vi "SetRGB.vi"(0 "ColorRGBA in":refnum<class "ColorRGBA.lvclass">, 5 "R":u8, 7 "G":u8, 9 "B":u8, 11 "error in (no error)":errorcluster) -> (4 "ColorRGBA out":refnum<class "ColorRGBA.lvclass">, 15 "error out":errorcluster)   [LabVIEW 2021, in "Picture2D.lvlib" / "ColorRGBA.lvclass"]
uses:
  ColorRGBA.lvclass
  ColorRGB/ColorRGB.lvclass
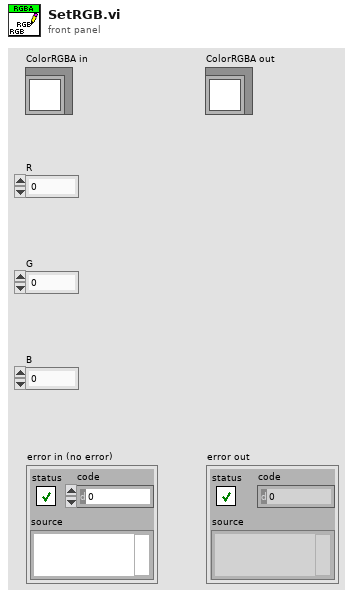
[diagram p1: front panel]
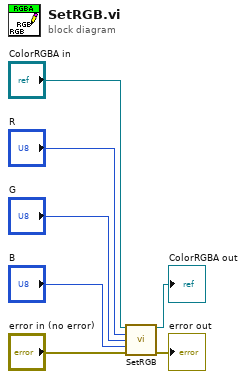
[diagram p0: block diagram]
diagram:
  n1 = call-parent "SetRGB.vi"("ColorRGB in"="ColorRGBA in", "R"="R", "G"="G", "B"="B", "error in (no error)"="error in (no error)") -> ("ColorRGB out"=→"ColorRGBA out":refnum<class "ColorRGBA.lvclass">, "error out"=→"error out":errorcluster)  [unwired: 9 in]
